vi "Cluster_2.vi"() -> ()   [LabVIEW 2023]
panel:
  out "병아리반 토익 평균":dbl
  in  "병아리반":cluster{"이름":string, "토익성적":dbl, "성별":bool}[](array[cluster])
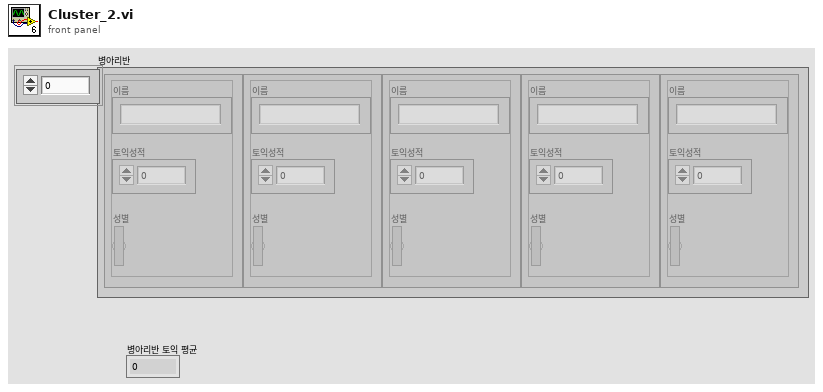
[diagram p1: front panel]
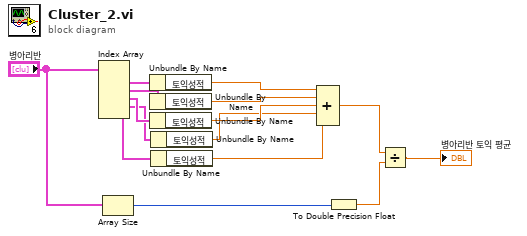
[diagram p0: block diagram]
diagram:
  n1 = Index Array(array="병아리반") -> (element #1=w15:cluster{"이름":string, "토익성적":dbl, "성별":bool}, element #2=w14:cluster{"이름":string, "토익성적":dbl, "성별":bool}, element #3=w13:cluster{"이름":string, "토익성적":dbl, "성별":bool}, element #4=w12:cluster{"이름":string, "토익성적":dbl, "성별":bool}, element #5=w11:cluster{"이름":string, "토익성적":dbl, "성별":bool})  [unwired: 5 in]
  n2 = Array Size(array="병아리반") -> (size(s)=w3:i32)
  n3 = Unbundle By Name(w15) -> ("토익성적"=w10:dbl)
  n4 = Unbundle By Name(w14) -> ("토익성적"=w9:dbl)
  n5 = Unbundle By Name(w13) -> ("토익성적"=w8:dbl)
  n6 = Unbundle By Name(w12) -> ("토익성적"=w7:dbl)
  n7 = Unbundle By Name(w11) -> ("토익성적"=w6:dbl)
  n8 = Compound Arithmetic op=ADD(w10, w9, w8, w7, w6) -> (w5:dbl)
  n9 = To Double Precision Float(number=w3) -> (double precision float=w2:dbl)
  n10 = Divide(x=w5, y=w2) -> (x/y=→"병아리반 토익 평균":dbl)
